vi "G4BaseTemplate_Singleton_6x8x6_SetProperty.vi"(2 "Property":dbl, 5 "error in (no error)":errorcluster) -> (19 "error out":errorcluster)   [LabVIEW 2018]
uses:
  <resource>/Framework/Providers/Open_GDS/ClassProviders/Provider_EndevoGOOP400/Templates/G4BaseTemplate_Singleton_6x8x6/G4BaseTemplate_Singleton_6x8x6.lvclass
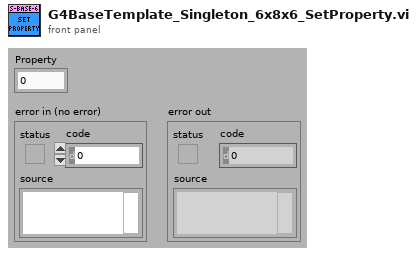
[diagram p1: front panel]
types:
  T1 = typedef "G4BaseTemplate_Singleton_6x8x6.lvclass/ObjectAttributes.ctl" = cluster{"Attribute1":dbl}
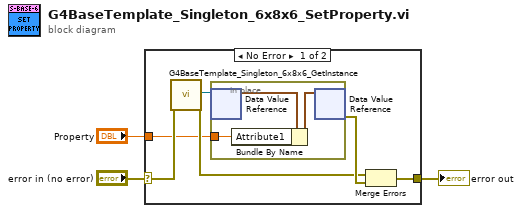
[diagram p0: block diagram]
diagram:
  n1 = case shown="No Error" "error in (no error)" {
    selector: "error in (no error)" -> [w9 w13]
    tunnel: [w6 w13] -> w2
    tunnel: "Property" -> [w4 _]
    frame No Error {
      n2 = call <resource>:"G4BaseTemplate_Singleton_6x8x6_GetInstance.vi"("error in (no error)"=w9) -> ("DVRRefOut"=w5:refnum<data-value>, "error out"=w7:errorcluster)  [unwired: 14 in, 3 out]
      n3 = in-place {
        in-place-border: w4 -> [w12]
        n4 = in-place-dvr #1(w5) -> (w11:T1)  [unwired: 1 out]
        n5 = Bundle By Name(cluster=w11, "Attribute1"=w12) -> (w10:T1)
        n6 = in-place-dvr #1(w10) -> (w8:errorcluster)  [unwired: 1 out]
      }
      n7 = Merge Errors(w7, w8) -> (w6:errorcluster)
    }
    frame Error {
    }
  }
  "error out" <- w2
